vi "Property Node.vi"() -> ()   [LabVIEW 2014]
panel:
  in  "stop":bool
  out "Vertical Progress Bar":u8(slide) scale=0.0..10.0
  in  "Knob":dbl(knob) scale=0.0..10.0
  out "led":bool
  in  "Button":bool
  # "PROPERTY NODE"
  # "BUTTON"
  # "LED"
  # "KNOB"
  # "PB"
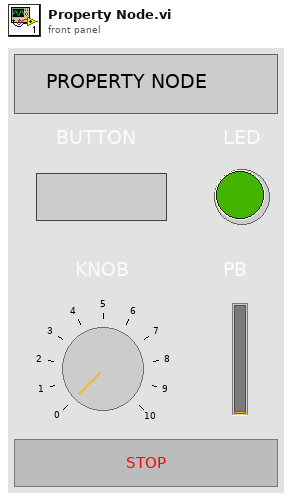
[diagram p1: front panel]
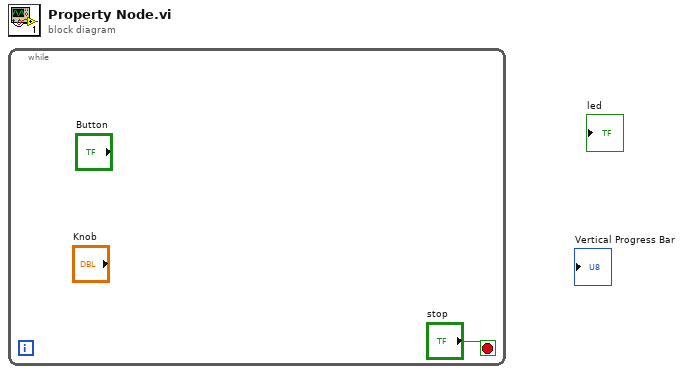
[diagram p0: block diagram]
diagram:
  n1 = while {
    stop <- "stop" stop-if-true
  }
